vi "GetMenuItems.vi"(8 "error in (no error)":errorcluster, 11 "ModeCol in":refnum<class "ModeCol.lvclass">) -> (0 "error out":errorcluster, 1 "LMenu tags":string[](array[string])=["Continue", "Ramp"], 2 "LMenu names":string[](array[string])=["Continue", "Ramp"], 3 "ModeCol out":refnum<class "ModeCol.lvclass">)   [LabVIEW 2013, in "ModeCol.lvclass"]
uses:
  ModeCol.lvclass
  ModeCol.lvclass/ModeCol.ctl
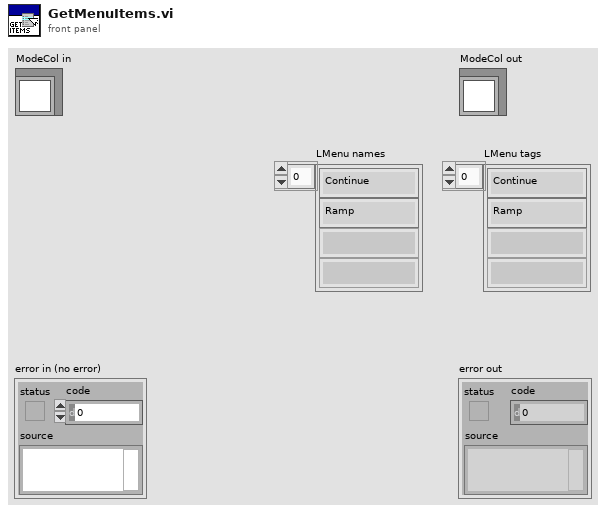
[diagram p1: front panel]
types:
  T1 = cluster{"Mode":string, "ModeTag":string, "Disables?":bool}[]
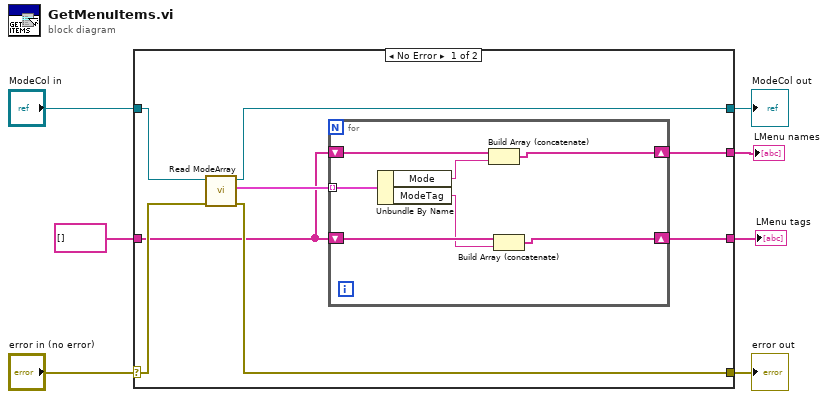
[diagram p0: block diagram]
diagram:
  n1 = case shown="No Error" "error in (no error)" {
    selector: "error in (no error)" -> [w13 w25]
    tunnel: [w12 w25] -> w6
    tunnel: [w14 w24] -> w4
    tunnel: "ModeCol in" -> [w15 w24]
    tunnel: [w10 w23] -> w3
    tunnel: [w9 w23] -> w2
    tunnel: string[] [] -> [w8 w23]
    frame No Error {
      n2 = call "Read ModeArray.vi"("error in (no error)"=w13, "ModeCol in"=w15) -> ("error out"=w12:errorcluster, "Array"=w11:T1, "ModeCol out"=w14:refnum<class "ModeCol.lvclass">)  [unwired: 7 in]
      n3 = for {
        tunnel: w11 -> [w22] mode=indexing
        shift-right: [w19] -> w10
        shift-left: w8 -> [w21]
        shift-right: [w17] -> w9
        shift-left: w8 -> [w18]
        n4 = Unbundle By Name(w22) -> ("Mode"=w20:string, "ModeTag"=w16:string)
        n5 = Build Array (concatenate)(w21, w20) -> (w19:string[])
        n6 = Build Array (concatenate)(w18, w16) -> (w17:string[])
      }
    }
    frame Error {
    }
  }
  "error out" <- w6
  "ModeCol out" <- w4
  "LMenu tags" <- w2
  "LMenu names" <- w3
